vi "CheckIfComposition.vi"(8 "error in (no error)":errorcluster, 11 "SMO.UI.MAUI in":refnum<class "SMO.UI.MAUI.lvclass">) -> (0 "error out":errorcluster, 2 "Is Composition?":bool, 3 "SMO.UI.MAUI out":refnum<class "SMO.UI.MAUI.lvclass">)   [LabVIEW 2020, in "SMO.UI.MAUI.lvclass"]
uses:
  SMO.UI.MAUI.lvclass
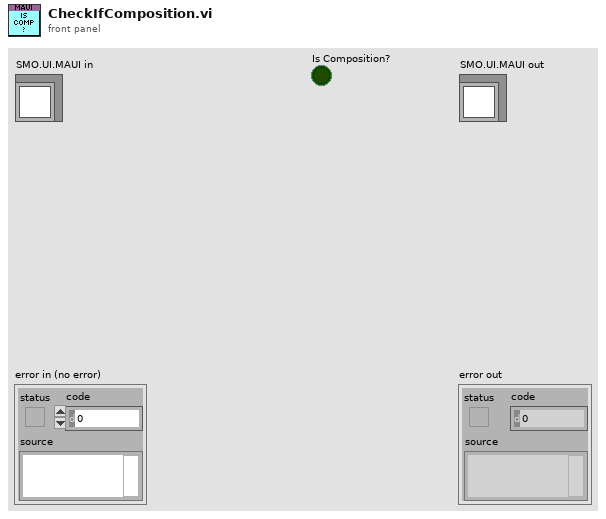
[diagram p1: front panel]
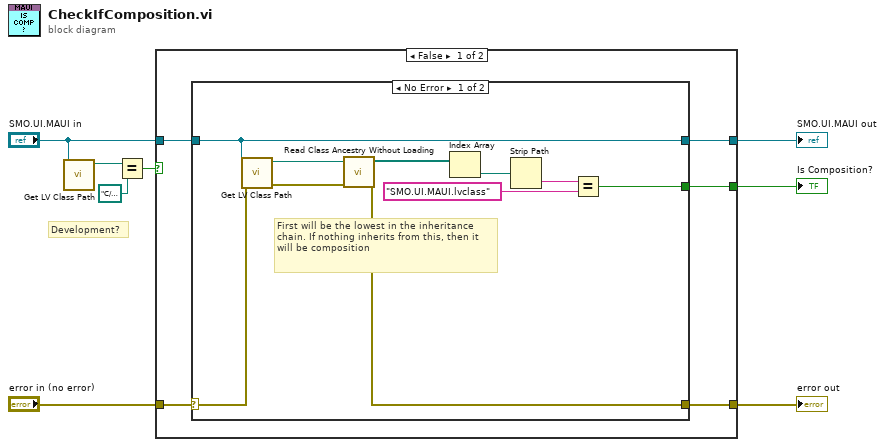
[diagram p0: block diagram]
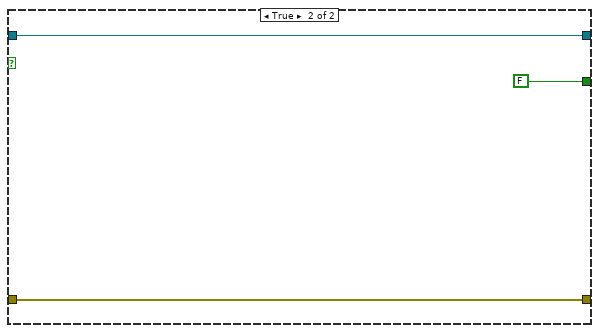
[diagram p3: hidden frame]
diagram:
  # "Development?"
  n1 = call <vilib>:"Get LV Class Path.vi"("object"="SMO.UI.MAUI in") -> ("class path"=w3:path)  [unwired: 9 in, 1 out]
  n2 = Equal?(x=w3, y=path "C:/Users/monke/Documents/GitHub/MAUI-Engine/lvsrc/SMO.UI.MAUI.lvclass") -> (x = y?=w1:bool)
  n3 = case shown="False" w1 {
    tunnel: "error in (no error)" -> [w13 w27]
    tunnel: [w12 w27] -> w7
    tunnel: "SMO.UI.MAUI in" -> [w11 w28]
    tunnel: [w10 w28] -> w6
    tunnel: [w9 FALSE] -> w5
    frame False {
      n4 = case shown="No Error" w13 {
        selector: w13 -> [w16 w25]
        tunnel: [w15 w25] -> w12
        tunnel: [w23 w24] -> w10
        tunnel: w11 -> [w23 w24]
        tunnel: [w14 _] -> w9
        frame No Error {
          # "First will be the lowest in the inheritance chain. If nothing inherits from this, then it will be composition"
          n5 = call <vilib>:"Get LV Class Path.vi"("error in (no error)"=w16, "object"=w23) -> ("error out"=w21:errorcluster, "class path"=w22:path)  [unwired: 8 in]
          n6 = call <vilib>:"Read Class Ancestry Without Loading.vi"("error in (no error)"=w21, "LabVIEW Class Path"=w22) -> ("error out"=w15:errorcluster, "Class Ancestry"=w20:path[])  [unwired: 8 in]
          n7 = Index Array(array=w20) -> (element=w19:path)  [unwired: 1 in]
          n8 = Strip Path(path=w19) -> (name=w18:string)  [unwired: 1 out]
          n9 = Equal?(x=w18, y="SMO.UI.MAUI.lvclass") -> (x = y?=w14:bool)
        }
        frame Error {
        }
      }
    }
    frame True {
    }
  }
  "error out" <- w7
  "SMO.UI.MAUI out" <- w6
  "Is Composition?" <- w5
